vi "extractTaslRefTerminal.vi"(8 "error in (no error)":errorcluster, 11 "VI in":refnum<vi>) -> (0 "error out":errorcluster, 1 "found?":bool, 2 "taskRefTerminal":refnum<vi>, 3 "VI out":refnum<vi>)   [LabVIEW 2023]
uses:
  <vilib>/Utility/traverseref.llb/TRef TravTarget.ctl
  <vilib>/Utility/traverseref.llb/VI Scripting - Traverse.lvlib
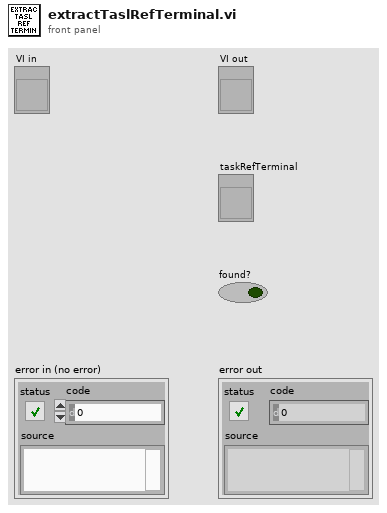
[diagram p1: front panel]
types:
  T1 = typedef "TRef TravTarget.ctl" = enum16{"FP", "BD", "Other"}
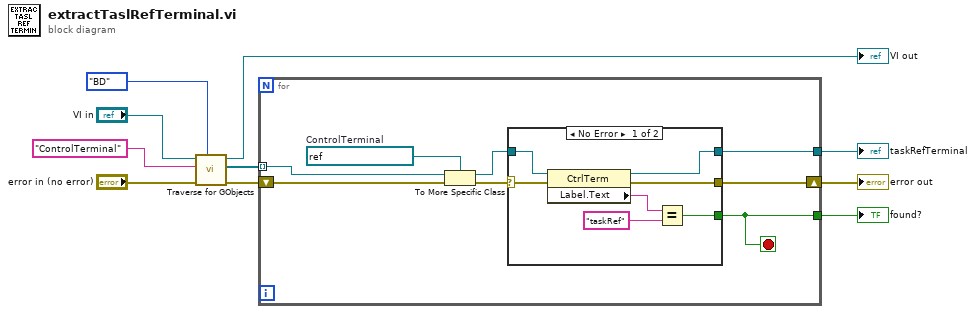
[diagram p0: block diagram]
diagram:
  n1 = call <vilib>:"Traverse for GObjects.vi"("Traverse Target"=TRef_TravTarget."BD", "error in (no error)"="error in (no error)", "Class Name"="ControlTerminal", "VI Refnum"="VI in") -> ("error out"=w6:errorcluster, "References"=w10:refnum<vi>[], "dup VI Refnum"=→"VI out":refnum<vi>)  [unwired: 4 in, 1 out]
  n2 = for {
    tunnel: w10 -> [w11] mode=indexing
    shift-right: [w14] -> w7
    shift-left: w6 -> [w15]
    tunnel: [w13] -> w9
    tunnel: [w12] -> w8
    stop <- w12 stop-if-true
    w16 = refnum<vi> refnum  # ControlTerminal
    n3 = To More Specific Class(target class=w16, reference=w11, error in=w15) -> (specific class reference=w17:refnum<vi>, error out=w18:errorcluster)
    n4 = case shown="No Error" w18 {
      selector: w18 -> [w25 _]
      tunnel: w17 -> [w24 _]
      tunnel: [w23 _] -> w14
      tunnel: [w20 _] -> w12
      tunnel: [w19 _] -> w13
      frame No Error {
        n5 = property class="CtrlTerm"(reference=w24, error in=w25) -> (reference out=w19:refnum<vi>, error out=w23:errorcluster, "Label.Text"=w22:string)
        n6 = Equal?(x=w22, y="taskRef") -> (x = y?=w20:bool)
      }
      frame Error {
      }
    }
  }
  "taskRefTerminal" <- w9
  "found?" <- w8
  "error out" <- w7
